vi "升立德IO写输出.vi"(0 "IO输出":T1, 3 "error in (no error)":errorcluster caption="错误输入（无错误）") -> (6 "IO输出":T1, 7 "结果":bool, 9 "error out":errorcluster caption="错误输出")   [LabVIEW 2014]
uses:
  IOoutput.ctl
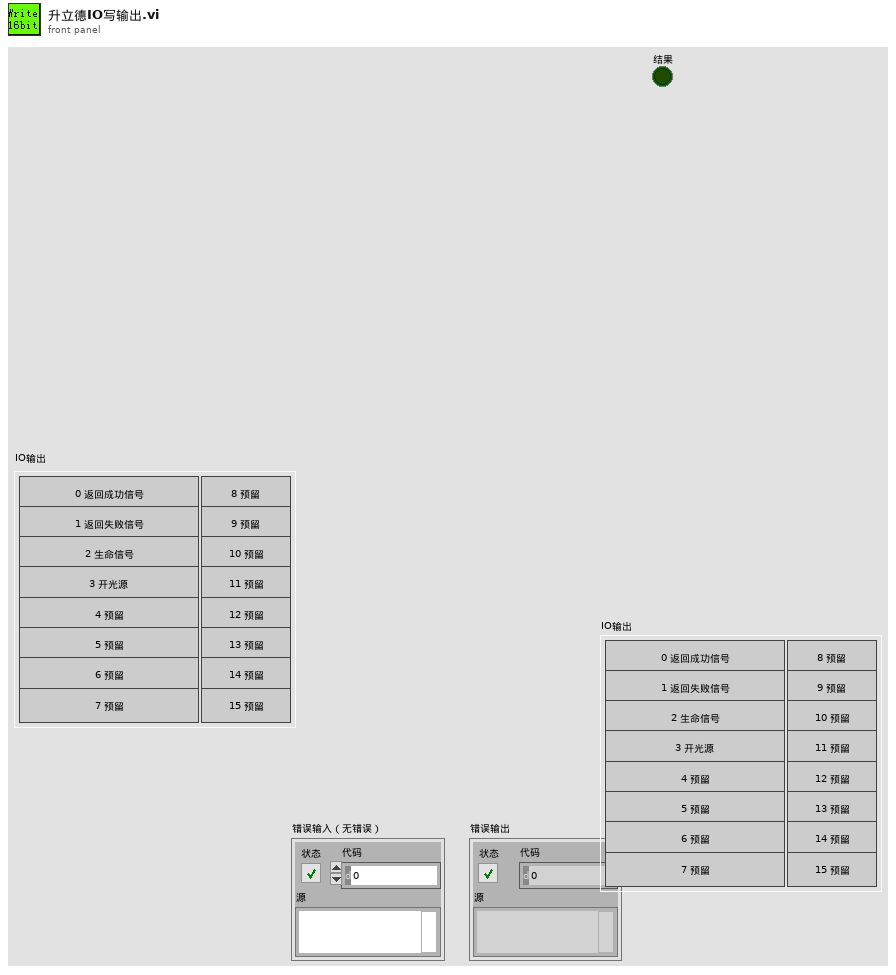
[diagram p1: front panel]
types:
  T1 = typedef "IOoutput.ctl" = cluster{"0 返回成功信号":bool, "1 返回失败信号":bool, "2 生命信号":bool, "3 开光源":bool, "4 预留":bool, "5 预留":bool, "6 预留":bool, "7 预留":bool, "8 预留":bool, "9 预留":bool, "10 预留":bool, "11 预留":bool, "12 预留":bool, "13 预留":bool, "14 预留":bool, "15 预留":bool}
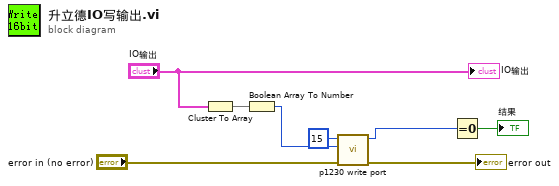
[diagram p0: block diagram]
diagram:
  n1 = Cluster To Array(cluster="IO输出") -> (array=w5:bool[])
  n2 = Boolean Array To Number(Boolean array=w5) -> (number=w4:u32)
  n3 = call "p1230 write port.vi"("error in (no error)"="error in (no error)", "data"=w4, "board_id"=u32 15) -> ("error out"=→"error out":errorcluster, "function return"=w2:u32)  [unwired: 7 in]
  n4 = Equal To 0?(x=w2) -> (x = 0?=→"结果":bool)
  "IO输出" <- "IO输出"
